vi "BuildModbusURLs.vi"(8 "error in":errorcluster, 10 "Chassis Num":i32, 11 "Chassis Cfg":refnum<class "ChassisCfg.lvclass">) -> (0 "error out":errorcluster, 3 "Chassis Cfg":refnum<class "ChassisCfg.lvclass">)   [LabVIEW 2012, in "Configuration Grandmaster.lvlib" / "ChassisCfg.lvclass"]
uses:
  ChassisCfg.lvclass
  ChassisCfg.lvclass/ChassisCfg.ctl
  Common/Controls/TE_Designator.ctl
  Class Timing Group/TimingGrp.lvclass
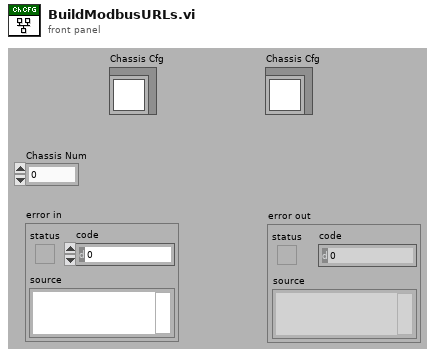
[diagram p1: front panel]
types:
  T1 = typedef "TE_Designator.ctl" = enum16{"High Speed", "Low Speed"}
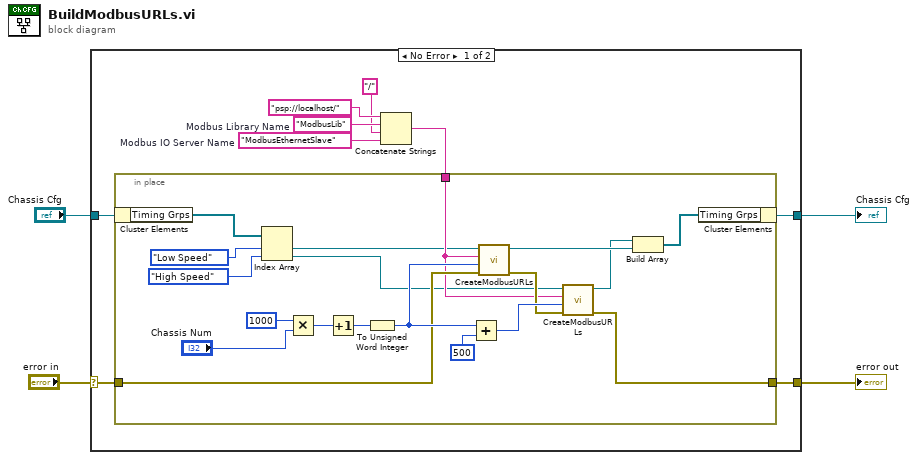
[diagram p0: block diagram]
diagram:
  n1 = case shown="No Error" "error in" {
    selector: "error in" -> [w9 w34]
    tunnel: "Chassis Cfg" -> [w6 w33]
    tunnel: [w5 w33] -> w3
    tunnel: [w8 w34] -> w1
    frame No Error {
      w13 = "ModbusEthernetSlave"  # Modbus IO Server Name
      w12 = "ModbusLib"  # Modbus Library Name
      n2 = Concatenate Strings("psp://localhost/", w12, "/" ("string"), w13) -> (w7:string)
      n3 = in-place {
        in-place-border: w9 -> [w25]
        in-place-border: [w23] -> w8
        in-place-border: w7 -> [w22]
        n4 = in-place-cluster #1(w6) -> ("Timing Grps"=w15:refnum<class "TimingGrp.lvclass">[])
        n5 = Index Array(array=w15, index #1=TE_Designator."Low Speed" ("Timing Engine"), index #2=TE_Designator."High Speed" ("Timing Engine")) -> (element #1=w19:refnum<class "TimingGrp.lvclass">, element #2=w18:refnum<class "TimingGrp.lvclass">)
        n6 = Multiply(x=1000, y="Chassis Num") -> (x*y=w31:i32)
        n7 = Increment(x=w31) -> (x+1=w29:i32)
        n8 = To Unsigned Word Integer(number=w29) -> (unsigned 16bit integer=w26:u16)
        n9 = Add(x=w26, y=u16 500) -> (x+y=w27:u16)
        n10 = call "CreateModbusURLs.vi"("error in (no error)"=w25, "Start Address"=w26, "Base Addres URL"=w22, "Timing Groups"=w19) -> ("error out"=w24:errorcluster, "Timing Groups"=w17:refnum<class "TimingGrp.lvclass">)  [unwired: 6 in]
        n11 = call "CreateModbusURLs.vi"("error in (no error)"=w24, "Start Address"=w27, "Base Addres URL"=w22, "Timing Groups"=w18) -> ("error out"=w23:errorcluster, "Timing Groups"=w16:refnum<class "TimingGrp.lvclass">)  [unwired: 6 in]
        n12 = Build Array(w16, w17) -> (w14:refnum<class "TimingGrp.lvclass">[])
        n13 = in-place-cluster #1("Timing Grps"=w14) -> (w5:refnum<class "ChassisCfg.lvclass">)
      }
    }
    frame Error {
    }
  }
  "error out" <- w1
  "Chassis Cfg" <- w3
